vi "Array Panel Async.vi"(10 "Container":refnum<vi>, 11 "PanelArray in":refnum<class "ArrayManager.lvclass">) -> ()   [LabVIEW 2020, in "OOPanel.lvlib" / "ArrayManager.lvclass"]
uses:
  ArrayManager.lvclass
  UI State.ctl
  ArrayManager.lvclass/ArrayManager.ctl
  ArrayPanel/ArrayPanel.lvclass
panel:
  out "Page Size":dbl
  in  "Scrollbar":i32(c297)
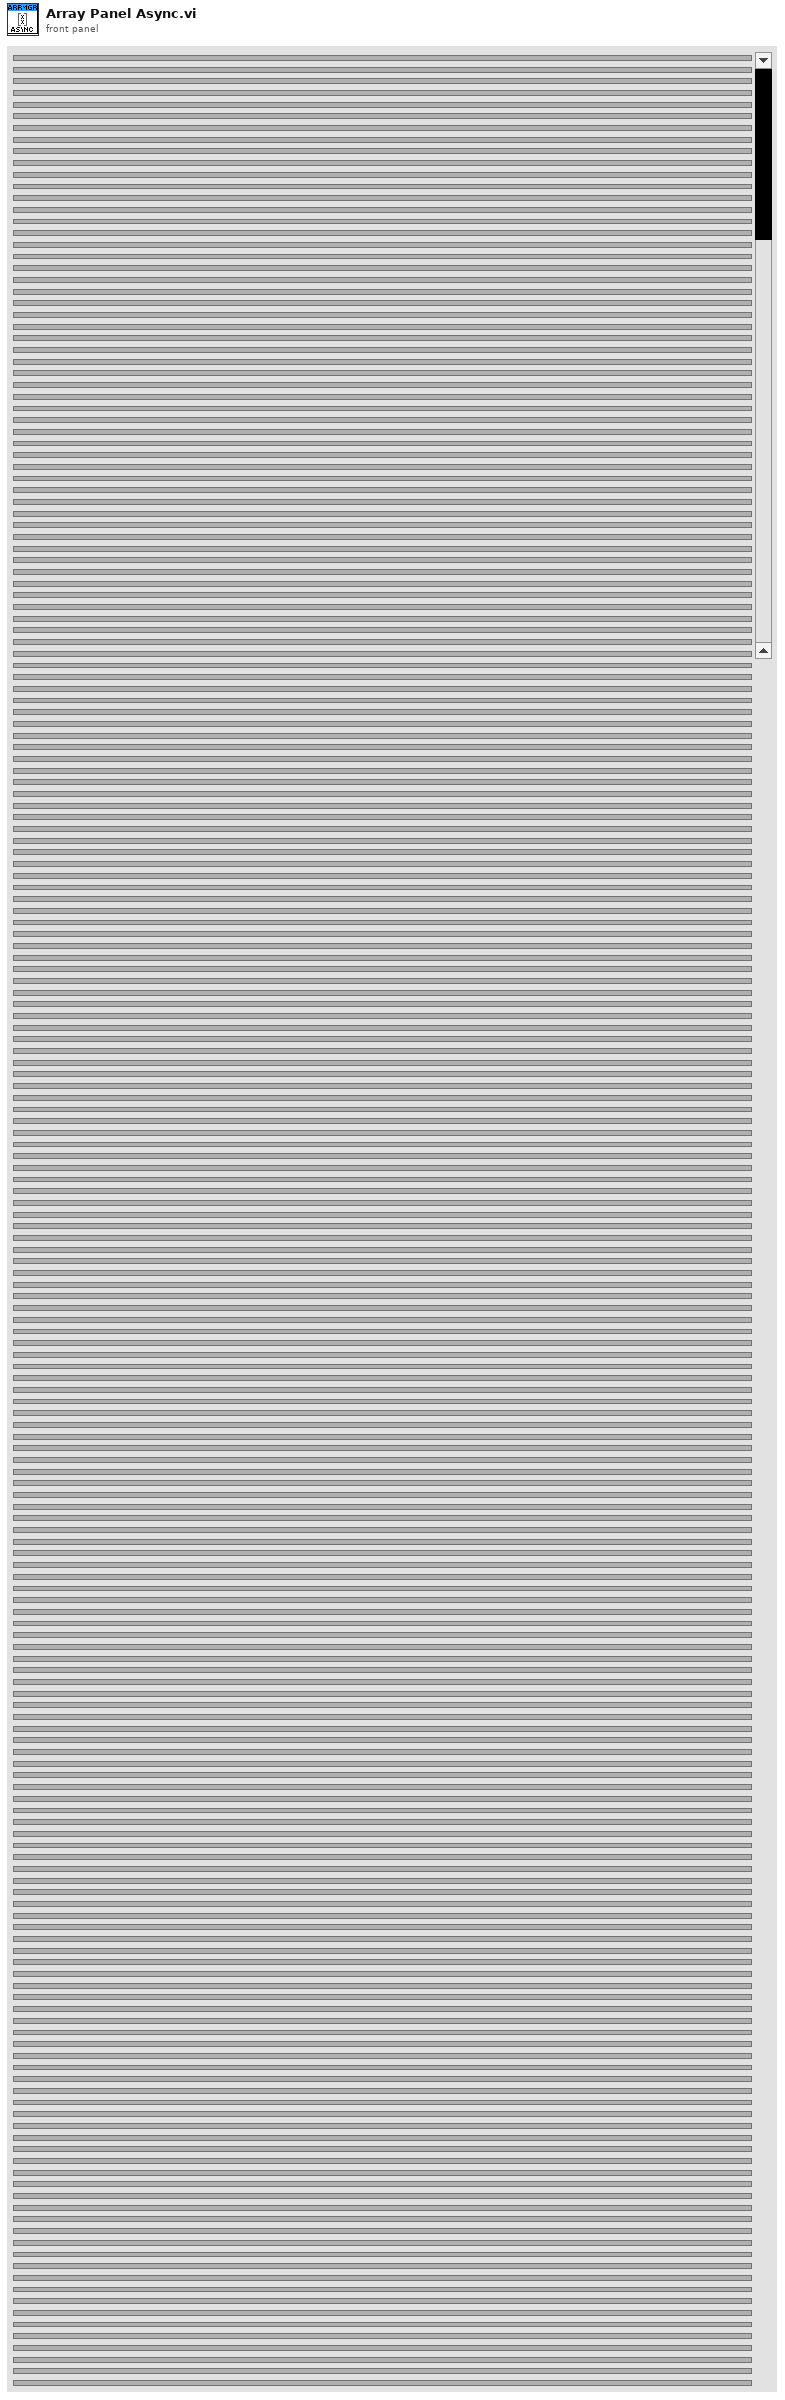
[diagram p1: front panel]
types:
  T1 = typedef "OOPanel.lvlib/ArrayManager.lvclass/UI State.ctl" = enum16{"Init", "Run", "Close"}
  T2 = typedef "OOPanel.lvlib/ArrayManager.lvclass/State Ref.ctl" = cluster{"Running":bool, "Borders":bool, "Total Height":dbl, "Scroll Visible":bool, "Background":u32}
  T3 = typedef "OOPanel.lvlib/ArrayManager.lvclass/UI Refs.ctl" = cluster{"SubPanels":refnum<vi>[], "Scrollbar":refnum<vi>, "Panel VI":refnum<vi>, "Container":refnum<vi>}
  T4 = typedef "OOPanel.lvlib/ArrayManager.lvclass/Events.ctl" = cluster{"Stop":refnum<user-event>, "Update":refnum<user-event>, "Scroll":refnum<user-event>, "Set BG":refnum<user-event>, "Scroll To Panel":refnum<user-event>}
  T5 = typedef "OOPanel.lvlib/Desired Size.ctl" = cluster{"Width":u32, "Height":u32}
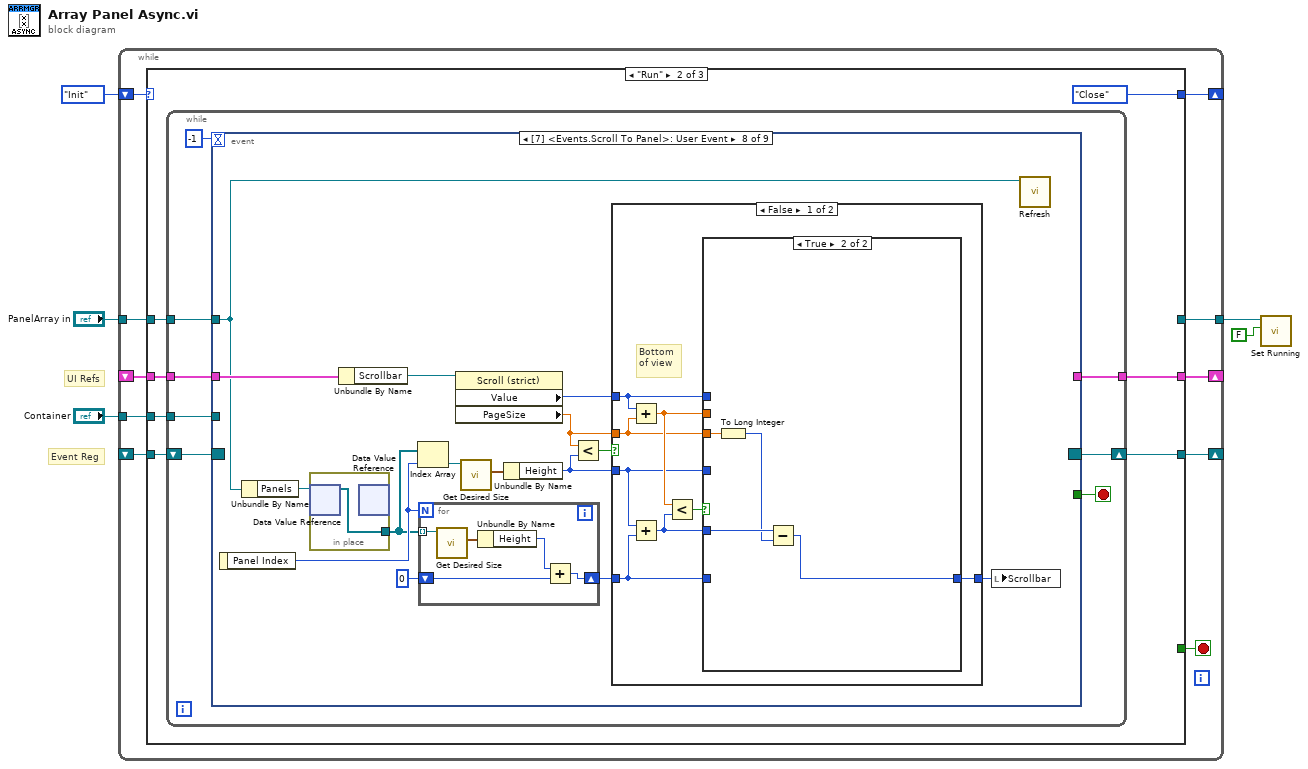
[diagram p0: block diagram]
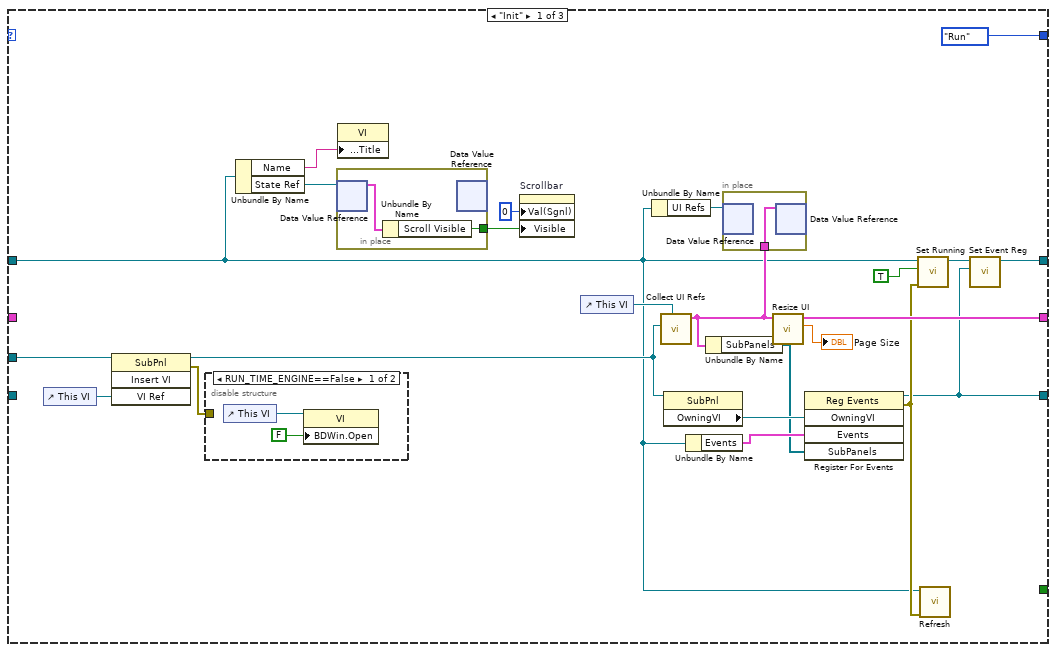
[diagram p2: hidden frame]
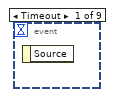
[diagram p4: hidden frame]
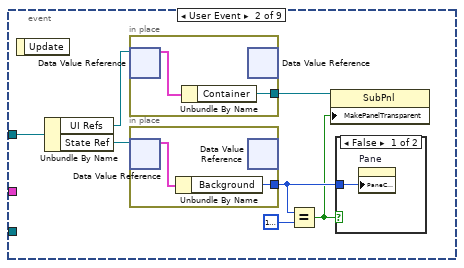
[diagram p5: hidden frame]
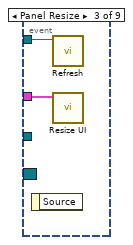
[diagram p7: hidden frame]
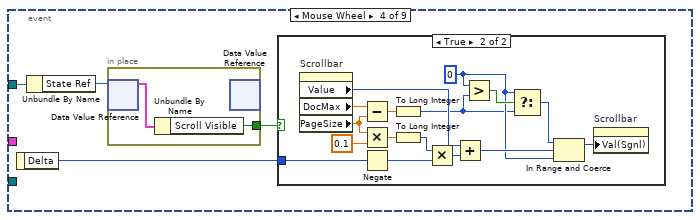
[diagram p8: hidden frame]
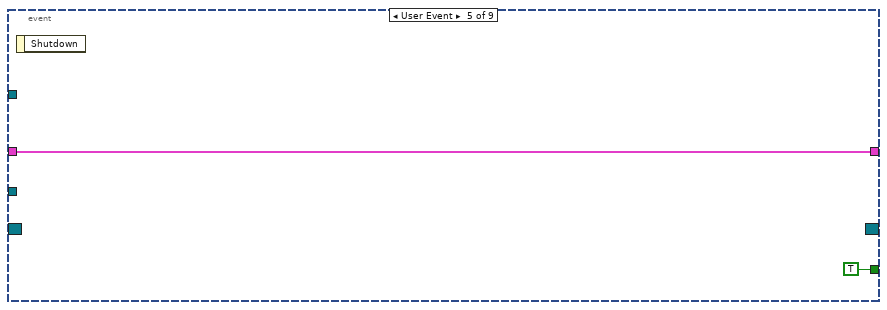
[diagram p10: hidden frame]
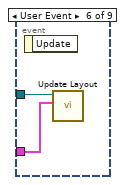
[diagram p11: hidden frame]
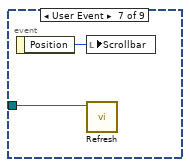
[diagram p12: hidden frame]
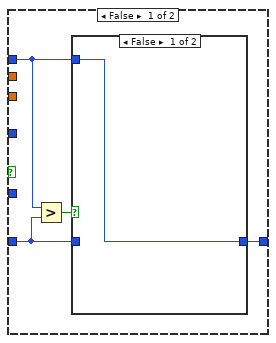
[diagram p13: hidden frame]
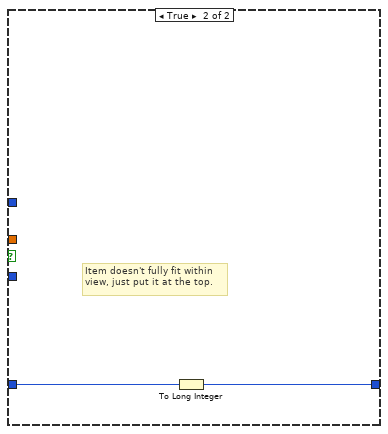
[diagram p15: hidden frame]
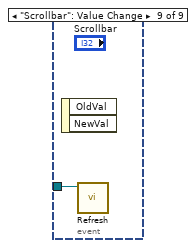
[diagram p16: hidden frame]
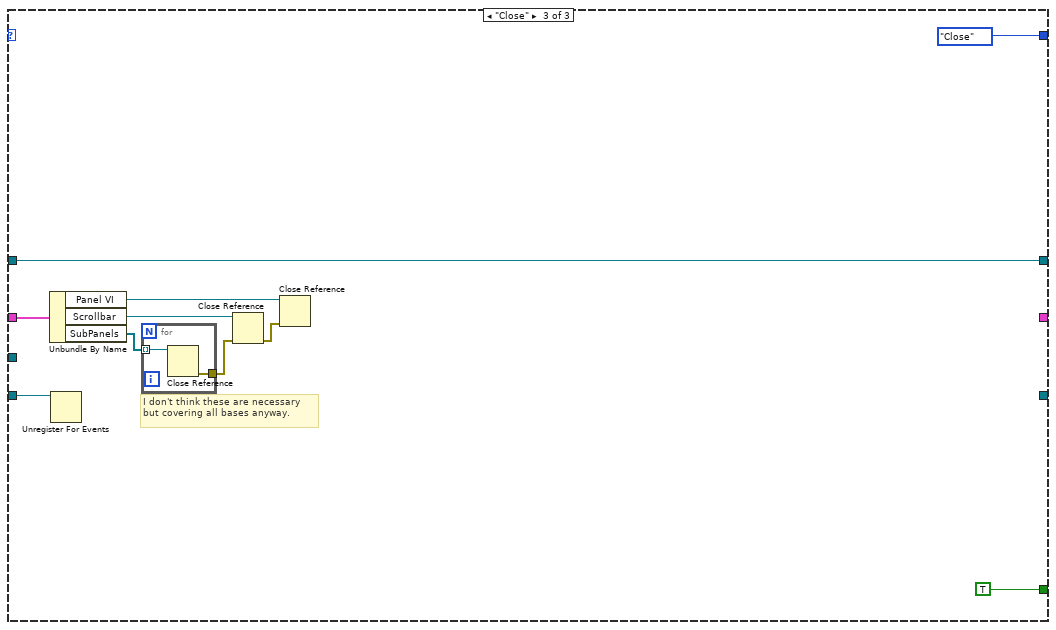
[diagram p17: hidden frame]
diagram:
  # "Event Reg"
  # "UI Refs"
  n1 = while {
    shift-right: [w14] -> _
    shift-left: UI_State."Init" ("UI State") -> [w15]
    tunnel: "PanelArray in" -> [w13]
    tunnel: "Container" -> [w11]
    shift-right: [w10] -> _
    shift-left: _ -> [w9]
    shift-right: [w8] -> _
    shift-left: _ -> [w7]
    tunnel: [w6] -> w2
    stop <- w12 stop-if-true
    n2 = case shown="\"Run\"" w15 {
      tunnel: [UI_State."Run" ("UI State") UI_State."Close" ("UI State") UI_State."Close" ("UI State")] -> w14
      tunnel: w13 -> [w16 w49 w143]
      tunnel: [_ _ TRUE] -> w12
      tunnel: w11 -> [w31 w48 _]
      tunnel: [w18 w47 _] -> w10
      tunnel: w9 -> [_ w46 w150]
      tunnel: [w34 w44 _] -> w8
      tunnel: w7 -> [_ w45 w149]
      tunnel: [w19 _ w143] -> w6
      frame "Init" {
        n3 = control-ref of="This VI"() -> (w30:refnum<vi>)
        n4 = invoke class="SubPnl" method="Insert VI"(reference=w31, "VI Ref"=w30) -> (reference out=w29:refnum<vi>, error out=w28:errorcluster)  [unwired: 2 in, 2 out]
        n5 = disable-structure shown="RUN_TIME_ENGINE==False" {
          disable-tunnel: w28 -> [_ _]
          frame condition #0 (active) {
            n6 = control-ref of="This VI"() -> (w43:refnum<vi>)
            n7 = property class="VI"(reference=w43, "BDWin.Open"=FALSE ("Block Diagram Window:Open")) -> ()  [unwired: 1 in, 2 out]
          }
          frame condition #1 {
          }
        }
        n8 = Unbundle By Name(w16) -> ("Name"=w17:string, "State Ref"=w25:refnum<data-value>)
        n9 = in-place {
          in-place-border: [w40] -> w24
          n10 = in-place-dvr #1(w25) -> (w41:T2)  [unwired: 1 out]
          n11 = Unbundle By Name(w41) -> ("Scroll Visible"=w40:bool)
          n12 = in-place-dvr #1() -> ()  [unwired: 1 in, 2 out]
        }
        n13 = property class="VI"("Front Panel.Title"=w17) -> ()  [unwired: 2 in, 2 out]
        n14 = property on="Scrollbar" class="Scroll (strict)"("Val(Sgnl)"=0 ("Value (Signaling)"), "Visible"=w24) -> ()  [unwired: 2 in, 2 out]
        n15 = control-ref of="This VI"() -> (w37:refnum<vi>)
        n16 = Unbundle By Name(w16) -> ("UI Refs"=w23:refnum<data-value>)
        n17 = call "Collect UI Refs.vi"("VI Refnum"=w37, "Container"=w29) -> ("UI Refs"=w22:T3)  [unwired: 9 in]
        n18 = property class="SubPnl"(reference=w29) -> ("OwningVI"=w35:refnum<vi>)  [unwired: 1 in, 2 out]
        n19 = Unbundle By Name(w16) -> ("Events"=w33:T4)
        n20 = Unbundle By Name(w22) -> ("SubPanels"=w26:refnum<vi>[])
        n21 = in-place {
          in-place-border: w22 -> [w39]
          n22 = in-place-dvr #2(w23) -> ()  [unwired: 2 out]
          n23 = in-place-dvr #2(w39) -> ()  [unwired: 2 out]
        }
        n24 = call "Resize UI.vi"("UI Refs In"=w22) -> ("Page Size"=→"Page Size":dbl, "UI Refs"=w34:T3)  [unwired: 9 in]
        n25 = register-events(w35, w33, w26) -> (reference out=w18:refnum<event-registration>, error out=w21:errorcluster)  [unwired: 2 in]
        n26 = call "Set Running.vi"("error in (no error)"=w21, "Running"=TRUE, "ArrayManager in"=w16) -> ("ArrayManager out"=w20:refnum<class "ArrayManager.lvclass">)  [unwired: 7 in, 1 out]
        n27 = call "Refresh.vi"("error in (no error)"=w21, "ArrayManager in"=w16) -> ()  [unwired: 8 in, 2 out]
        n28 = call "Set Event Reg.vi"("Event Reg"=w18, "ArrayManager in"=w20) -> ("ArrayManager out"=w19:refnum<class "ArrayManager.lvclass">)  [unwired: 8 in, 1 out]
      }
      frame "Run" {
        n29 = while {
          tunnel: w49 -> [w57]
          tunnel: w48 -> [w56]
          shift-right: [w55] -> w47
          shift-left: w46 -> [w54]
          tunnel: w45 -> [w53]
          tunnel: [w52] -> w44
          stop <- w51 stop-if-true
          n30 = event shown="[7] <Events.Scroll To Panel>: User Event" {
            selector: w54 -> [_ _ _ _ _ _ _ _ _]
            dyn-events: [_ _ _ _ _ _ _ _ _] -> w55
            timeout: -1 -> [_ _ _ _ _ _ _ _ _]
            tunnel: w57 -> [_ w64 w71 w74 _ w98 w99 w105 w142]
            tunnel: w56 -> [_ _ _ _ _ _ _ _ _]
            tunnel: w53 -> [_ _ w72 _ w96 w97 _ w109 _]
            tunnel: [_ _ _ _ w96 _ _ _ _] -> w52
            tunnel: [_ _ _ _ TRUE _ _ _ _] -> w51
            event Timeout {
              n31 = event-data() -> ()  [unwired: 1 in, 1 out]
            }
            event User Event {
              n32 = event-data() -> ()  [unwired: 1 in, 1 out]
              n33 = Unbundle By Name(w64) -> ("UI Refs"=w61:refnum<data-value>, "State Ref"=w65:refnum<data-value>)
              n34 = in-place {
                in-place-border: [w66] -> w60
                n35 = in-place-dvr #3(w61) -> (w67:T3)  [unwired: 1 out]
                n36 = Unbundle By Name(w67) -> ("Container"=w66:refnum<vi>)
                n37 = in-place-dvr #3() -> ()  [unwired: 1 in, 2 out]
              }
              n38 = in-place {
                in-place-border: [w69] -> w62
                n39 = in-place-dvr #4(w65) -> (w70:T2)  [unwired: 1 out]
                n40 = Unbundle By Name(w70) -> ("Background"=w69:u32)
                n41 = in-place-dvr #4() -> ()  [unwired: 1 in, 2 out]
              }
              n42 = Equal?(x=w62, y=u32 16777216) -> (x = y?=w59:bool)
              n43 = property class="SubPnl"(reference=w60, "MakePanelTransparent"=w59) -> ()  [unwired: 1 in, 2 out]
              n44 = case shown="False" w59 {
                tunnel: w62 -> [w68 _]
                frame False {
                  n45 = property on="Pane" class="Pane"("PaneColor"=w68) -> ()  [unwired: 2 in, 2 out]
                }
                frame True {
                }
              }
            }
            event Panel Resize {
              n46 = event-data() -> ()  [unwired: 1 in, 1 out]
              n47 = call "Refresh.vi"("ArrayManager in"=w71) -> ()  [unwired: 9 in, 2 out]
              n48 = call "Resize UI.vi"("UI Refs In"=w72) -> ()  [unwired: 9 in, 2 out]
            }
            event Mouse Wheel {
              n49 = event-data() -> ("Delta"=w76:i32)  [unwired: 1 in]
              n50 = Unbundle By Name(w74) -> ("State Ref"=w75:refnum<data-value>)
              n51 = in-place {
                in-place-border: [w77] -> w73
                n52 = in-place-dvr #5(w75) -> (w78:T2)  [unwired: 1 out]
                n53 = Unbundle By Name(w78) -> ("Scroll Visible"=w77:bool)
                n54 = in-place-dvr #5() -> ()  [unwired: 1 in, 2 out]
              }
              n55 = case shown="True" w73 {
                tunnel: w76 -> [_ w79]
                frame False {
                }
                frame True {
                  w82 = 0 ("lower limit")
                  n56 = property on="Scrollbar" class="Scroll (strict)"() -> ("Value"=w90:i32, "DocMax"=w88:dbl, "PageSize"=w87:dbl)  [unwired: 2 in, 2 out]
                  n57 = Subtract(x=w88, y=w87) -> (x-y=w86:dbl)
                  n58 = Multiply(x=w87, y=0.1) -> (x*y=w93:dbl)
                  n59 = Negate(x=w79) -> (-x=w84:i32)
                  n60 = To Long Integer(number=w86) -> (32bit integer=w81:i32)
                  n61 = To Long Integer(number=w93) -> (32bit integer=w91:i32)
                  n62 = Multiply(x=w91, y=w84) -> (x*y=w92:i32)
                  n63 = Add(x=w90, y=w92) -> (x+y=w89:i32)
                  n64 = Greater?(x=w82, y=w81) -> (0:w83:bool)
                  n65 = Select(t=w82, s=w83, f=w81) -> (s? t:f=w80:i32)
                  n66 = In Range and Coerce(upper limit=w80, x=w89, lower limit=w82) -> (coerced(x)=w85:i32)  [unwired: 1 out]
                  n67 = property on="Scrollbar" class="Scroll (strict)"("Val(Sgnl)"=w85) -> ()  [unwired: 2 in, 2 out]
                }
              }
            }
            event User Event {
              n68 = event-data() -> ()  [unwired: 1 in, 1 out]
            }
            event User Event {
              n69 = event-data() -> ()  [unwired: 1 in, 1 out]
              n70 = call "Update Layout.vi"("UI Refs"=w97, "ArrayManager in"=w98) -> ()  [unwired: 8 in, 2 out]
            }
            event User Event {
              n71 = event-data() -> ("Position"=w100:i32)  [unwired: 1 in]
              n72 = local write "Scrollbar"(w100) -> ()
              n73 = call "Refresh.vi"("ArrayManager in"=w99) -> ()  [unwired: 9 in, 2 out]
            }
            event User Event {
              n74 = event-data() -> ("Panel Index"=w113:i32)  [unwired: 1 in]
              n75 = Unbundle By Name(w105) -> ("Panels"=w115:refnum<data-value>)
              n76 = in-place {
                in-place-border: [w141] -> w112
                n77 = in-place-dvr #6(w115) -> (w141:refnum<class "ArrayPanel.lvclass">[])  [unwired: 1 out]
                n78 = in-place-dvr #6() -> ()  [unwired: 1 in, 2 out]
              }
              n79 = Unbundle By Name(w109) -> ("Scrollbar"=w108:refnum<vi>)
              n80 = Index Array(array=w112, index=w113) -> (element=w111:refnum<class "ArrayPanel.lvclass">)
              n81 = for {
                N: w113 -> [_]
                tunnel: w112 -> [w140] mode=indexing
                shift-right: [w137] -> w106
                shift-left: u32 0 ("Height") -> [w138]
                n82 = call-dynamic "Get Desired Size.vi"("ArrayPanel in"=w140) -> ("Desired Size"=w139:T5)  [unwired: 8 in, 2 out]
                n83 = Unbundle By Name(w139) -> ("Height"=w136:u32)
                n84 = Add(x=w136, y=w138) -> (x+y=w137:u32)
              }
              n85 = property class="Scroll (strict)"(reference=w108) -> ("Value"=w101:i32, "PageSize"=w102:dbl)  [unwired: 1 in, 2 out]
              n86 = call-dynamic "Get Desired Size.vi"("ArrayPanel in"=w111) -> ("Desired Size"=w110:T5)  [unwired: 8 in, 2 out]
              n87 = Unbundle By Name(w110) -> ("Height"=w103:u32)
              n88 = Less?(x=w102, y=w103) -> (x < y?=w107:bool)
              n89 = case shown="False" w107 {
                tunnel: w106 -> [w122 w135]
                tunnel: [w120 w134] -> w104
                tunnel: w103 -> [w118 _]
                tunnel: w102 -> [w116 _]
                tunnel: w101 -> [w119 _]
                frame False {
                  # "Bottom of view"
                  n90 = Add(x=w119, y=w116) -> (x+y=w121:dbl)
                  n91 = Add(x=w118, y=w122) -> (x+y=w117:u32)
                  n92 = Less?(x=w121, y=w117) -> (x < y?=w123:bool)
                  n93 = case shown="True" w123 {
                    tunnel: w122 -> [w124 _]
                    tunnel: w121 -> [_ _]
                    tunnel: [w125 w131] -> w120
                    tunnel: w119 -> [w126 _]
                    tunnel: w118 -> [_ _]
                    tunnel: w117 -> [_ w133]
                    tunnel: w116 -> [_ w132]
                    frame False {
                      n94 = Greater?(x=w126, y=w124) -> (0:w127:bool)
                      n95 = case shown="False" w127 {
                        tunnel: w126 -> [w128 _]
                        tunnel: [w128 w129] -> w125
                        tunnel: w124 -> [_ w129]
                        frame False {
                        }
                        frame True {
                        }
                      }
                    }
                    frame True {
                      n96 = To Long Integer(number=w132) -> (32bit integer=w130:i32)
                      n97 = Subtract(x=w133, y=w130) -> (x-y=w131:u32)
                    }
                  }
                }
                frame True {
                  # "Item doesn't fully fit within view, just put it at the top."
                  n98 = To Long Integer(number=w135) -> (32bit integer=w134:i32)
                }
              }
              n99 = local write "Scrollbar"(w104) -> ()
              n100 = call "Refresh.vi"("ArrayManager in"=w105) -> ()  [unwired: 9 in, 2 out]
            }
            event "Scrollbar": Value Change {
              n101 = event-data() -> ()  [unwired: 1 in, 2 out]
              n102 = call "Refresh.vi"("ArrayManager in"=w142) -> ()  [unwired: 9 in, 2 out]
            }
          }
        }
      }
      frame "Close" {
        # "I don't think these are necessary but covering all bases anyway."
        n103 = Unbundle By Name(w149) -> ("Panel VI"=w147:refnum<vi>, "Scrollbar"=w148:refnum<vi>, "SubPanels"=w145:refnum<vi>[])
        n104 = Unregister For Events(event registration refnum=w150) -> ()  [unwired: 1 in, 1 out]
        n105 = for {
          tunnel: w145 -> [w154] mode=indexing
          tunnel: [w153] -> w144
          n106 = Close Reference(reference=w154) -> (error out=w153:errorcluster)  [unwired: 1 in]
        }
        n107 = Close Reference(reference=w148, error in (no error)=w144) -> (error out=w146:errorcluster)
        n108 = Close Reference(reference=w147, error in (no error)=w146) -> ()  [unwired: 1 out]
      }
    }
  }
  n109 = call "Set Running.vi"("Running"=FALSE, "ArrayManager in"=w2) -> ()  [unwired: 8 in, 2 out]
